vi "sub_BFnBT.vi"(8 "error in":errorcluster caption="에러 입력(에러 없음)", 11 "wf sum in":waveform(dbl) caption="sum of wf") -> (0 "error out":errorcluster caption="에러 출력")   [LabVIEW 2013]
uses:
  <vilib>/Waveform/WDTOps.llb/WDT Waveform Duration DBL.vi
  <vilib>/measure/mamon.llb/Trigger Detection for 1 Channel.vi
  <vilib>/Waveform/WDTOps.llb/WDT Get Waveform Subset DBL.vi
  <vilib>/measure/mascope.llb/Amplitude and Levels 1 chan.vi
  <vilib>/measure/NI_MAPro.lvlib
panel:
  out "P_time":dbl
  out "Pickup graph":waveform(dbl)(graph)
  out "P_force":dbl format="%.2p"
  out "B_time":dbl
  out "B_force":dbl format="%.2p"
  out "Bonding graph":waveform(dbl)(graph)
  out "wf":waveform(dbl)(graph)
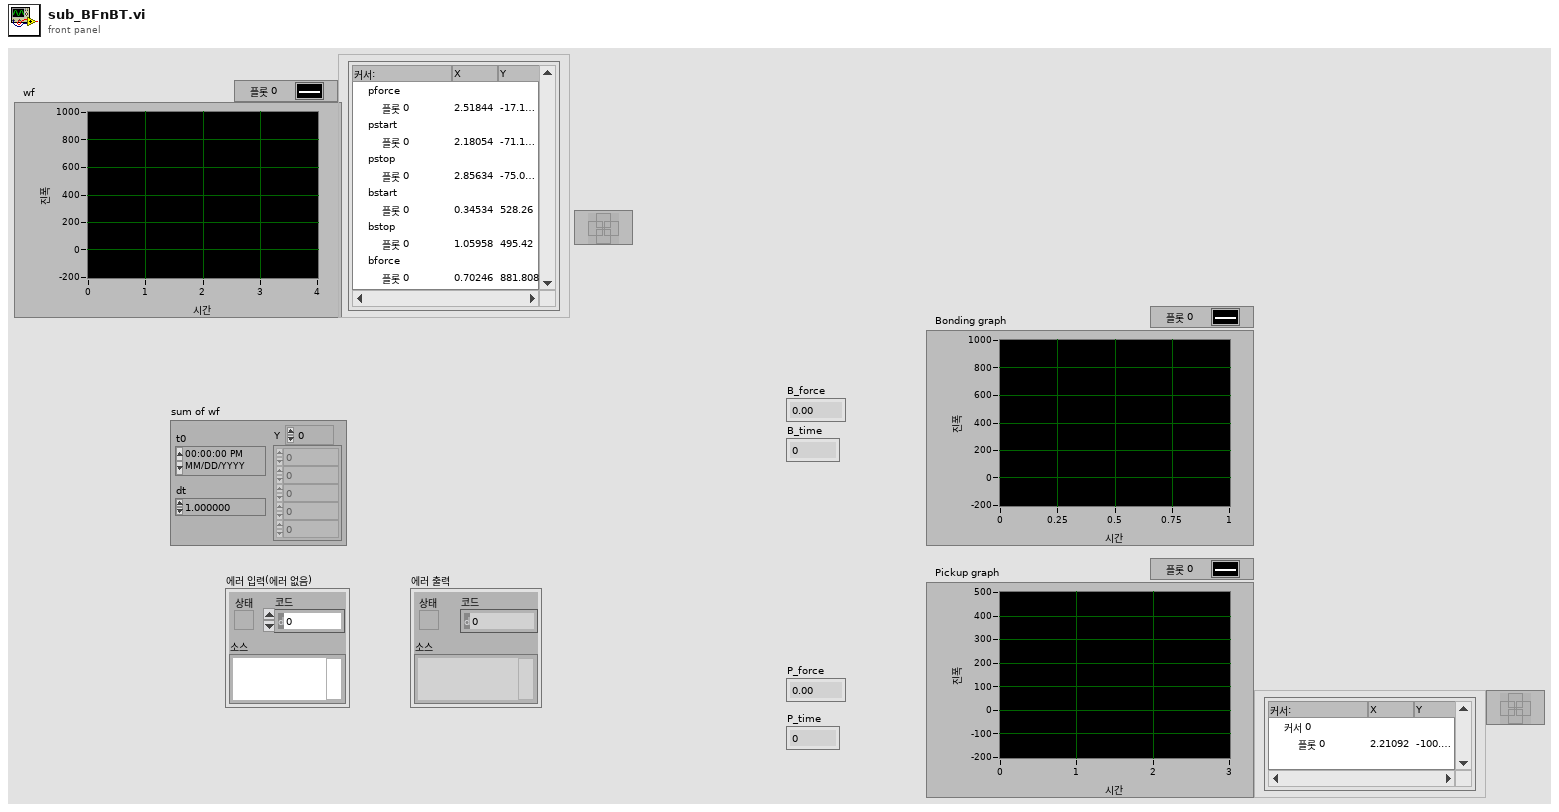
[diagram p1: front panel]
types:
  T1 = typedef "config_ctl.ctl" = cluster{"Trigger minlevel":dbl, "Lower Cut-Off":dbl, "Force high_level":dbl, "state settings":cluster{"method":enum32{"histogram", "peak", "auto select"}, "histogram size":i32, "histogram method":enum16{"mode"}, "reserved":dbl}, "SPA-300 Setting":cluster{"Bonding force (g)":dbl, "Bonding time (ms)":dbl, "Pickup force (g)":dbl, "Pickup time (ms)":dbl, "Speed":enum16{"Slow", "Fast"}}}
  T2 = typedef "UI_ctl.ctl" = cluster{"vacuum 차트":refnum<vi>, "vacuum":refnum<vi>, "Strain raw graph":refnum<vi>, "Strain raw chart":refnum<vi>, "Bonding time":refnum<vi>, "Bonding force":refnum<vi>, "Balance":refnum<vi>, "Filtered force graph":refnum<vi>, "ROI intensity":refnum<vi>, "Heater_rt":refnum<vi>, "Tensile force":refnum<vi>}
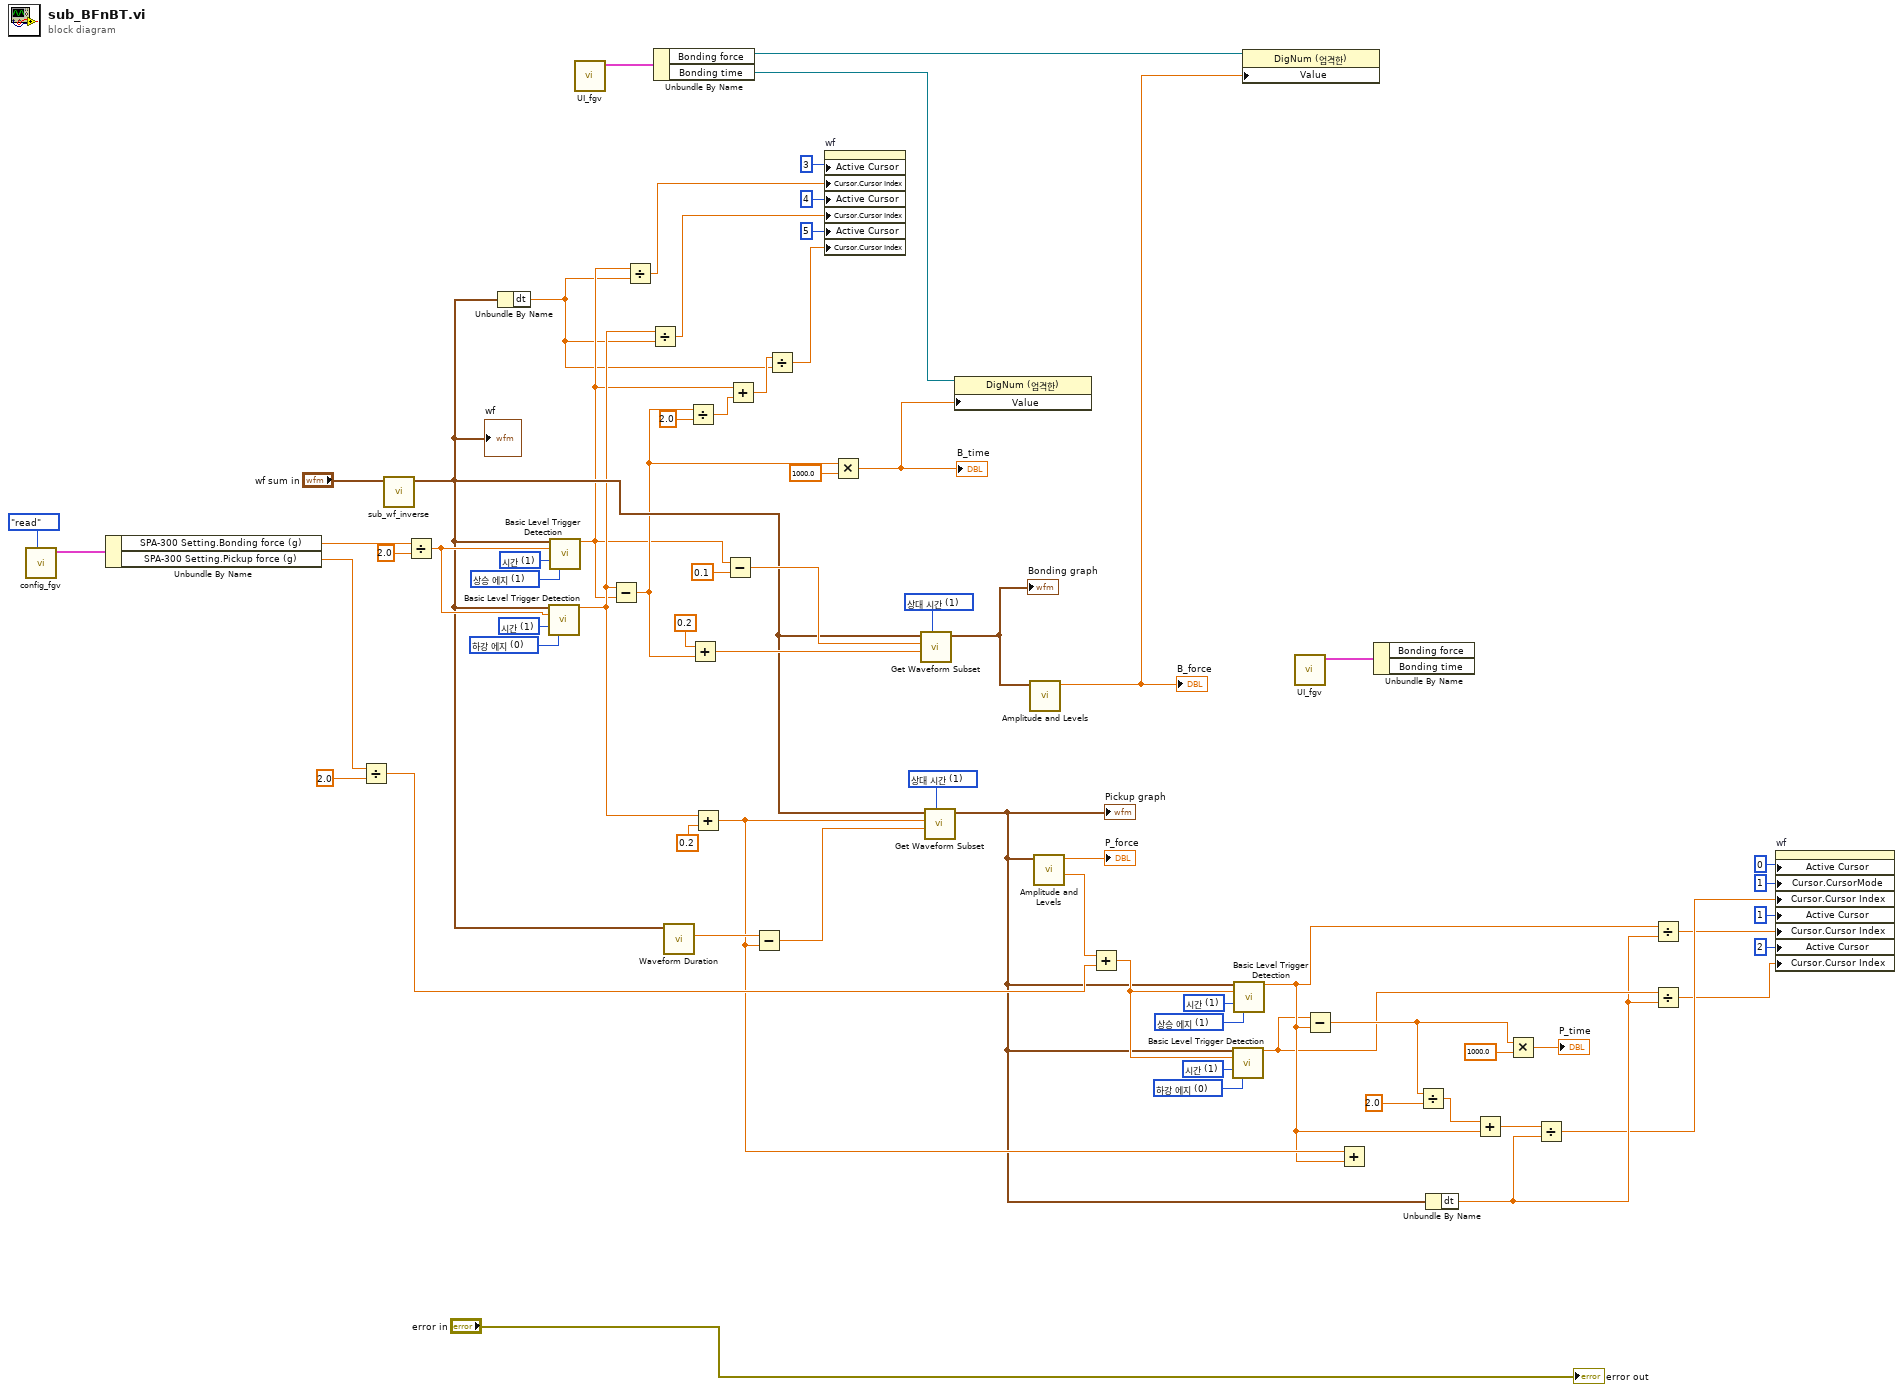
[diagram p0: block diagram]
diagram:
  w45 = u16 0 items=["하강 에지", "상승 에지"] ("trigger slope")
  w44 = u16 1 items=["인덱스", "시간"] ("location mode")
  w43 = u16 1 items=["하강 에지", "상승 에지"] ("trigger slope")
  w42 = u16 1 items=["인덱스", "시간"] ("location mode")
  w51 = u16 1 items=["샘플 ", "상대 시간"] ("start/duration format")
  w57 = u16 1 items=["샘플 ", "상대 시간"] ("start/duration format")
  w60 = u16 0 items=["하강 에지", "상승 에지"] ("trigger slope")
  w61 = u16 1 items=["인덱스", "시간"] ("location mode")
  w62 = u16 1 items=["하강 에지", "상승 에지"] ("trigger slope")
  w63 = u16 1 items=["인덱스", "시간"] ("location mode")
  n1 = call "config_fgv.vi"("cmd"=enum16{"write", "read", "ini"}."read") -> ("Config out"=w68:T1)  [unwired: 9 in, 1 out]
  n2 = Unbundle By Name(w68) -> ("SPA-300 Setting.Bonding force (g)"=w65:dbl, "SPA-300 Setting.Pickup force (g)"=w49:dbl)
  n3 = Divide(x=w49, y=2.0) -> (x/y=w39:dbl)
  n4 = call "sub_wf_inverse.vi"("Trigger graph"="wf sum in") -> ("inverse graph"=w14:waveform(dbl))  [unwired: 10 in]
  "wf" <- w14
  n5 = Divide(x=w65, y=2.0) -> (x/y=w41:dbl)
  n6 = Unbundle By Name(w14) -> ("dt"=w2:dbl)
  n7 = call-poly <vilib>:"Basic Level Trigger Detection.vi"("signal in"=w14, "level"=w41, "location mode"=w61, "trigger slope"=w60) -> ("trigger location"=w13:dbl)  [unwired: 9 in, 2 out]
  n8 = call-poly <vilib>:"Basic Level Trigger Detection.vi"("signal in"=w14, "level"=w41, "location mode"=w63, "trigger slope"=w62) -> ("trigger location"=w4:dbl)  [unwired: 9 in, 2 out]
  n9 = call "UI_fgv.vi"() -> ("UI cluster out"=w69:T2)  [unwired: 11 in]
  n10 = Subtract(x=w13, y=w4) -> (x-y=w7:dbl)
  n11 = Divide(x=w4, y=w2) -> (x/y=w9:dbl)
  n12 = Divide(x=w13, y=w2) -> (x/y=w8:dbl)
  n13 = Unbundle By Name(w69) -> ("Bonding force"=w70:refnum<vi>, "Bonding time"=w66:refnum<vi>)
  n14 = call-poly <vilib>:"Waveform Duration.vi"("waveform in"=w14) -> ("duration"=w47:dbl)  [unwired: 8 in, 2 out]
  n15 = Divide(x=w7, y=2.0) -> (x/y=w5:dbl)
  n16 = Add(x=0.2 ("y"), y=w7) -> (x+y=w54:dbl)
  n17 = Add(x=w13, y=0.2) -> (x+y=w30:dbl)
  n18 = Subtract(x=w4, y=0.1) -> (x-y=w56:dbl)
  n19 = Add(x=w4, y=w5) -> (x+y=w3:dbl)
  n20 = Subtract(x=w47, y=w30) -> (x-y=w46:dbl)
  n21 = Divide(x=w3, y=w2) -> (x/y=w1:dbl)
  n22 = property on="wf" class="WFGraph (엄격한)"("Active Cursor"=u32 3 ("활성 커서"), "Cursor.Cursor Index"=w9, "Active Cursor"=u32 4 ("활성 커서"), "Cursor.Cursor Index"=w8, "Active Cursor"=u32 5 ("활성 커서"), "Cursor.Cursor Index"=w1) -> ()  [unwired: 2 in, 2 out]
  n23 = Multiply(x=w7, y=1000.0) -> (x*y=w31:dbl)
  "B_time" <- w31
  n24 = call-poly <vilib>:"Get Waveform Subset.vi"("start/duration format"=w57, "duration"=w54, "start samples/time"=w56, "waveform in"=w14) -> ("waveform out"=w52:waveform(dbl))  [unwired: 2 in, 3 out]
  "Bonding graph" <- w52
  n25 = call-poly <vilib>:"Get Waveform Subset.vi"("start/duration format"=w51, "duration"=w46, "start samples/time"=w30, "waveform in"=w14) -> ("waveform out"=w24:waveform(dbl))  [unwired: 2 in, 3 out]
  "Pickup graph" <- w24
  n26 = property class="DigNum (엄격한)"(reference=w66, "Value"=w31) -> ()  [unwired: 1 in, 2 out]
  n27 = call-poly <vilib>:"Amplitude and Levels.vi"("signal in"=w52) -> ("amplitude"=w37:dbl)  [unwired: 7 in, 3 out]
  "B_force" <- w37
  n28 = call-poly <vilib>:"Amplitude and Levels.vi"("signal in"=w24) -> ("low state level"=w40:dbl, "amplitude"=→"P_force":dbl)  [unwired: 7 in, 2 out]
  n29 = Add(x=w40, y=w39) -> (x+y=w38:dbl)
  n30 = call-poly <vilib>:"Basic Level Trigger Detection.vi"("signal in"=w24, "level"=w38, "location mode"=w44, "trigger slope"=w45) -> ("trigger location"=w22:dbl)  [unwired: 9 in, 2 out]
  n31 = call-poly <vilib>:"Basic Level Trigger Detection.vi"("signal in"=w24, "level"=w38, "location mode"=w42, "trigger slope"=w43) -> ("trigger location"=w23:dbl)  [unwired: 9 in, 2 out]
  n32 = property class="DigNum (엄격한)"(reference=w70, "Value"=w37) -> ()  [unwired: 1 in, 2 out]
  n33 = call "UI_fgv.vi"() -> ("UI cluster out"=w36:T2)  [unwired: 11 in]
  n34 = Subtract(x=w22, y=w23) -> (x-y=w25:dbl)
  n35 = Add(x=w30, y=w23) -> ()  [unwired: 1 out]
  n36 = Unbundle By Name(w36) -> ()  [unwired: 2 out]
  n37 = Divide(x=w25, y=2.0) -> (x/y=w27:dbl)
  n38 = Unbundle By Name(w24) -> ("dt"=w21:dbl)
  n39 = Add(x=w27, y=w23) -> (x+y=w26:dbl)
  n40 = Multiply(x=w25, y=1000.0) -> (x*y=→"P_time":dbl)
  n41 = Divide(x=w26, y=w21) -> (x/y=w20:dbl)
  n42 = Divide(x=w23, y=w21) -> (x/y=w15:dbl)
  n43 = Divide(x=w22, y=w21) -> (x/y=w18:dbl)
  n44 = property on="wf" class="WFGraph (엄격한)"("Active Cursor"=u32 0 ("활성 커서"), "Cursor.CursorMode"=u32 1 ("커서.커서 모드"), "Cursor.Cursor Index"=w20, "Active Cursor"=u32 1 ("활성 커서"), "Cursor.Cursor Index"=w15, "Active Cursor"=u32 2 ("활성 커서"), "Cursor.Cursor Index"=w18) -> ()  [unwired: 2 in, 2 out]
  "error out" <- "error in"
